vi "Machs1-15-07-2017.vi"(0 "d0Mach1":fxp<+/-,18,18> format="%.16g", 1 "heizenMach1":bool, 2 "U_SPMach1":fxp<+/-,26,5> format="%.23g", 3 "->Register":u32, 5 "d1Mach1":fxp<+/-,21,21> format="%.16g", 7 "Warten(uSec)":u16=5000, 9 "d0Mach2":fxp<+/-,18,18> format="%.16g", 11 "d1Mach2":fxp<+/-,21,21> format="%.16g", 12 "heizenMach2":bool, 13 "U_SPMach2":fxp<+/-,26,5> format="%.23g") -> (4 "U_MWMach1":fxp<+/-,26,5> format="%.23g", 14 "Register->":u32, 15 "U_MWMach2":fxp<+/-,26,5> format="%.23g")   [LabVIEW 2017]
uses:
  <vilib>/rvi/FXPMathLib/FxpDiv/subVIs/nifxpmath_Div_SimConfig.ctl
  <vilib>/rvi/FXPMathLib/FxpSqrt/subVIs/nifxpmath_Sqrt_SimConfig.ctl
  <vilib>/fxp/LVFixedPointOverflowPolicyTypeDef.ctl
  <vilib>/rvi/FXPMathLib/FxpConvert/subVIs/nifxpmath_Convert_SimConfig.ctl
  <vilib>/fxp/LVFixedPointQuantizationPolicyTypeDef.ctl
  <vilib>/rvi/eio/common/nirviEmuTemplateMethod_errors.vi
  <vilib>/rvi/FXPMathLib/FxpDiv/simVIs/DllFxpDivTemp_sub.vi
  <vilib>/rvi/FXPMathLib/FxpSqrt/simVIs/DllSqrtTemp_sub.vi
  <vilib>/rvi/FXPMathLib/FxpConvert/simVIs/DllFxpConvertTemp_sub.vi
  <vilib>/eio/EIONode/EIONode.xnode
  <vilib>/rvi/FXPMathLib/FxpAdd/XNode/nifxpmath_Add.xnode
  <vilib>/rvi/FXPMathLib/FxpDiv/XNode/nifxpmath_Div.xnode
  <vilib>/rvi/FXPMathLib/FxpMul/XNode/nifxpmath_Multiplier.xnode
  <vilib>/rvi/FXPMathLib/FxpSqrt/XNode/nifxpmath_Sqrt.xnode
  <vilib>/rvi/FXPMathLib/FxpConvert/XNode/nifxpmath_Convert.xnode
  <vilib>/rvi/FXPMathLib/FxpSub/XNode/nifxpmath_Sub.xnode
  <vilib>/rvi/FXPMathLib/sim/FxpSim.dll
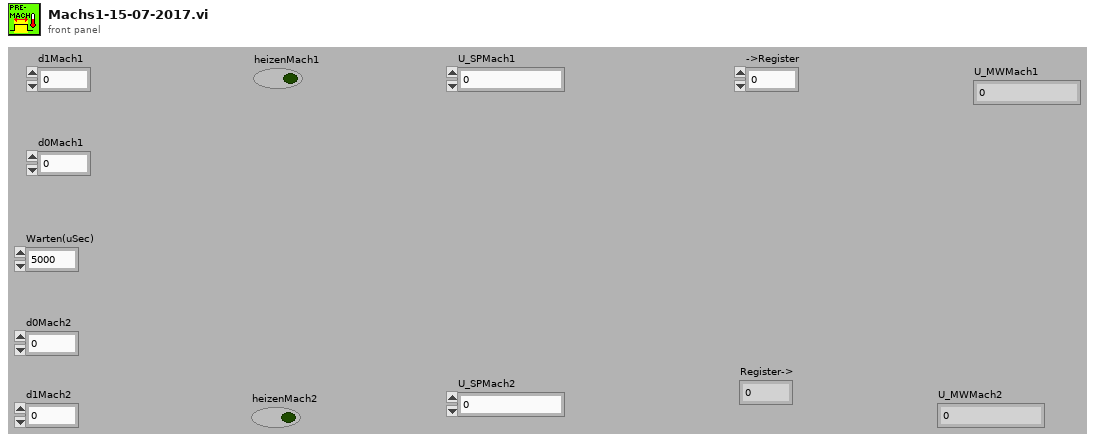
[diagram p1: front panel]
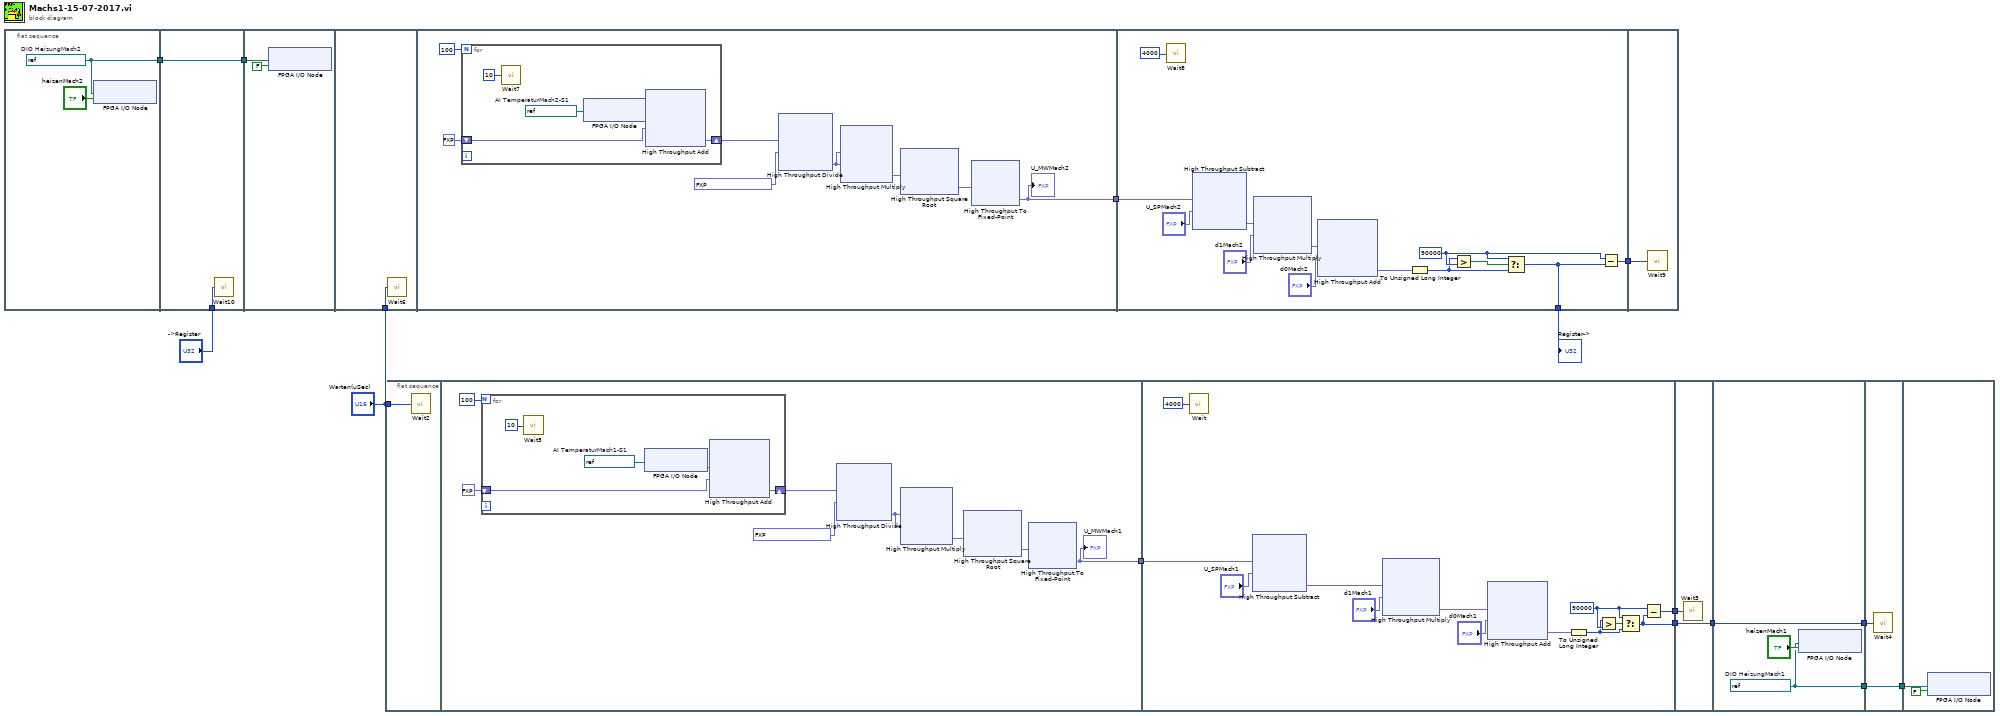
[diagram p0: block diagram]
diagram:
  n1 = flat-sequence {
    tunnel: [w15] -> w1
    tunnel: "->Register" -> [w18]
    tunnel: [w17] -> w2
    tunnel: w1 -> [w17]
    tunnel: w2 -> [w19]
    tunnel: "Warten(uSec)" -> [w21]
    tunnel: [w22] -> w8
    tunnel: w8 -> [w116]
    tunnel: [w110] -> w7
    tunnel: [w106] -> w6
    tunnel: w7 -> [w119]
    frame #0 {
      w15 = refnum<k21> "Mod6/DIO22"  # DIO HeizungMach2
      n2 = xnode "FPGA I/O Node"("I/O-Objekt"="heizenMach2", "FPGA-I/O (Eingang)"=w15) -> ()  [unwired: 1 out]
    }
    frame #1 {
      n3 = call "Wait10"("Count(uSec)"=w18) -> ()  [unwired: 1 out]
    }
    frame #2 {
      n4 = xnode "FPGA I/O Node"("I/O-Objekt"=FALSE ("I/O Item"), "FPGA-I/O (Eingang)"=w19) -> ()  [unwired: 1 out]
    }
    frame #3 {
      n5 = call "Wait6"("Count(uSec)"=w21) -> ()  [unwired: 1 out]
    }
    frame #4 {
      n6 = for {
        N: 100 -> [_]
        shift-right: [w102] -> w29
        shift-left: fxp<+/-,33,12> 0.0 ("x+y") -> [w103]
        w101 = refnum<k21> "Mod1/AI4"  # AI TemperaturMach2-S1
        n7 = call "Wait7"("Count(uSec)"=u8 10) -> ()  [unwired: 1 out]
        n8 = xnode "FPGA I/O Node"("FPGA-I/O (Eingang)"=w101) -> ("I/O-Objekt"=w104:fxp<+/-,26,5>)  [unwired: 1 out]
        n9 = xnode "High Throughput Add"("x"=w104, "y"=w103) -> ("x+y"=w102:fxp<+/-,33,12>)
      }
      n10 = xnode "High Throughput Divide"("x"=w29, "y"=fxp<+/-,8,8> 100.0) -> ("x/y"=w25:fxp<+/-,26,5>)
      n11 = xnode "High Throughput Multiply"("x"=w25, "y"=w25) -> ("x*y"=w24:fxp<+,52,10>)
      n12 = xnode "High Throughput Square Root"("x"=w24) -> ("sqrt(x)"=w23:fxp<+,26,5>)
      n13 = xnode "High Throughput To Fixed-Point"("x"=w23) -> ("y"=w22:fxp<+/-,26,5>)
      "U_MWMach2" <- w22
    }
    frame #5 {
      w108 = u32 90000 ("x")
      n14 = call "Wait8"("Count(uSec)"=u16 4000) -> ()  [unwired: 1 out]
      n15 = xnode "High Throughput Subtract"("x"=w116, "y"="U_SPMach2") -> ("x-y"=w115:fxp<+/-,26,5>)
      n16 = xnode "High Throughput Multiply"("x"=w115, "y"="d1Mach2") -> ("x*y"=w113:fxp<+/-,18,18>)
      n17 = xnode "High Throughput Add"("x"=w113, "y"="d0Mach2") -> ("x+y"=w111:fxp<+/-,18,18>)
      n18 = To Unsigned Long Integer(number=w111) -> (unsigned 32bit integer=w107:u32)
      n19 = Greater?(x=w107, y=w108) -> (0:w109:bool)
      n20 = Select(t=w108, s=w109, f=w107) -> (s? t:f=w106:u32)
      n21 = Subtract(x=w108, y=w106) -> (x-y=w110:u32)
    }
    frame #6 {
      n22 = call "Wait9"("Count(uSec)"=w119) -> ()  [unwired: 1 out]
    }
  }
  n23 = flat-sequence {
    tunnel: "Warten(uSec)" -> [w120]
    tunnel: [w121] -> w13
    tunnel: w13 -> [w215]
    tunnel: [w205] -> w12
    tunnel: [w209] -> w11
    tunnel: [w219] -> w10
    tunnel: w12 -> [w219]
    tunnel: w11 -> [w218]
    tunnel: [w221] -> w9
    tunnel: w10 -> [w221]
    tunnel: [w220] -> w3
    tunnel: w9 -> [w224]
    tunnel: [w223] -> w4
    tunnel: w3 -> [w223]
    tunnel: w4 -> [w225]
    frame #0 {
      n24 = call "Wait2"("Count(uSec)"=w120) -> ()  [unwired: 1 out]
    }
    frame #1 {
      n25 = for {
        N: 100 -> [_]
        shift-right: [w201] -> w128
        shift-left: fxp<+/-,33,12> 0.0 ("x+y") -> [w202]
        w200 = refnum<k21> "Mod1/AI3"  # AI TemperaturMach1-S1
        n26 = call "Wait5"("Count(uSec)"=u8 10) -> ()  [unwired: 1 out]
        n27 = xnode "FPGA I/O Node"("FPGA-I/O (Eingang)"=w200) -> ("I/O-Objekt"=w203:fxp<+/-,26,5>)  [unwired: 1 out]
        n28 = xnode "High Throughput Add"("x"=w203, "y"=w202) -> ("x+y"=w201:fxp<+/-,33,12>)
      }
      n29 = xnode "High Throughput Divide"("x"=w128, "y"=fxp<+/-,8,8> 100.0) -> ("x/y"=w124:fxp<+/-,26,5>)
      n30 = xnode "High Throughput Multiply"("x"=w124, "y"=w124) -> ("x*y"=w123:fxp<+,52,10>)
      n31 = xnode "High Throughput Square Root"("x"=w123) -> ("sqrt(x)"=w122:fxp<+,26,5>)
      n32 = xnode "High Throughput To Fixed-Point"("x"=w122) -> ("y"=w121:fxp<+/-,26,5>)
      "U_MWMach1" <- w121
    }
    frame #2 {
      w207 = u32 90000 ("x")
      n33 = call "Wait"("Count(uSec)"=u16 4000) -> ()  [unwired: 1 out]
      n34 = xnode "High Throughput Subtract"("x"=w215, "y"="U_SPMach1") -> ("x-y"=w214:fxp<+/-,26,5>)
      n35 = xnode "High Throughput Multiply"("x"=w214, "y"="d1Mach1") -> ("x*y"=w212:fxp<+/-,18,18>)
      n36 = xnode "High Throughput Add"("x"=w212, "y"="d0Mach1") -> ("x+y"=w210:fxp<+/-,18,18>)
      n37 = To Unsigned Long Integer(number=w210) -> (unsigned 32bit integer=w206:u32)
      n38 = Greater?(x=w206, y=w207) -> (0:w208:bool)
      n39 = Select(t=w207, s=w208, f=w206) -> (s? t:f=w205:u32)
      n40 = Subtract(x=w207, y=w205) -> (x-y=w209:u32)
    }
    frame #3 {
      n41 = call "Wait3"("Count(uSec)"=w218) -> ()  [unwired: 1 out]
    }
    frame #4 {
      w220 = refnum<k21> "Mod6/DIO23"  # DIO HeizungMach1
      n42 = xnode "FPGA I/O Node"("I/O-Objekt"="heizenMach1", "FPGA-I/O (Eingang)"=w220) -> ()  [unwired: 1 out]
    }
    frame #5 {
      n43 = call "Wait4"("Count(uSec)"=w224) -> ()  [unwired: 1 out]
    }
    frame #6 {
      n44 = xnode "FPGA I/O Node"("I/O-Objekt"=FALSE ("I/O Item"), "FPGA-I/O (Eingang)"=w225) -> ()  [unwired: 1 out]
    }
  }
  "Register->" <- w6
